vi "Keithley 2002 T-Coup Config.vi"(0 "GPIB address":string="16", 1 "reference (off:0)":u16(ring) items=["off", "set reference value"], 2 "reference value (degs)":dbl format="%^.2e", 3 "T-couple type (J:0)":u16(ring) items=["J thermocouples", "T thermocouples", "K thermocouples", "E thermocouples", "R thermocouples", "S thermocouples", "B thermocouples", "B thermocouples"], 4 "simulated temp. (degs)":dbl=23.0 min=0.0 max=323.0 format="%^.2e", 5 "integration time (0:auto)":u16(ring) items=["automatic", "automatic once", "set to minimum", "set to maximum", "set aperature value", "set NPLC value"], 6 "real coefficient":dbl=0.01 min=-0.09999 max=0.09999 format="%^.2e", 7 "integ. value":dbl=0.01667 format="%^.2e", 8 "real offset":dbl=0.01 min=-0.09999 max=0.09999 format="%^.2e", 9 "resolution (5.5 digits:4)":u16(ring)=4 items=["auto resolution", "auto resolution once", "3.5 digits", "4.5 digits", "5.5 digits", "6.5 digits"], 11 "error in":T1, 12 "digital filter (off:0)":u16(ring) items=["off", "auto filter", "auto filter once", "moving filter", "repeating filter"], 13 "dig. filter count":dbl=10.0 min=1.0 max=100.0 step=1.0 format="%^.2e", 14 "temp (celsius:0)":u16(ring) items=["Celsius", "Fahrenheit", "Kelvin"]) -> (15 "error out":T1)   [LabVIEW 2020]
doc: "This VI is used to configure the settings for the thermo-couple temperature measurements. The instrument can be in any mode when this VI is run. The settings will go into effect and the instrument will go into the Temperature mode."
panel:
  in  "R-junction #":dbl=1.0 min=1.0 max=5.0
  in  "R-junction type":bool=TRUE
  # "simulated\nreal"
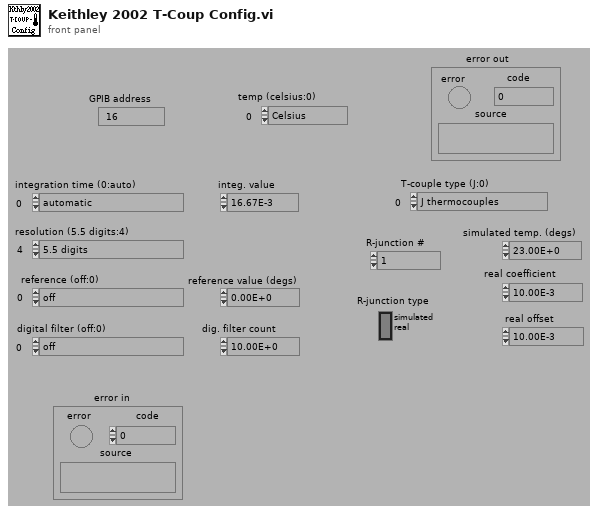
[diagram p1: front panel]
types:
  T1 = cluster{"error":bool, "code":i32, "source":string}
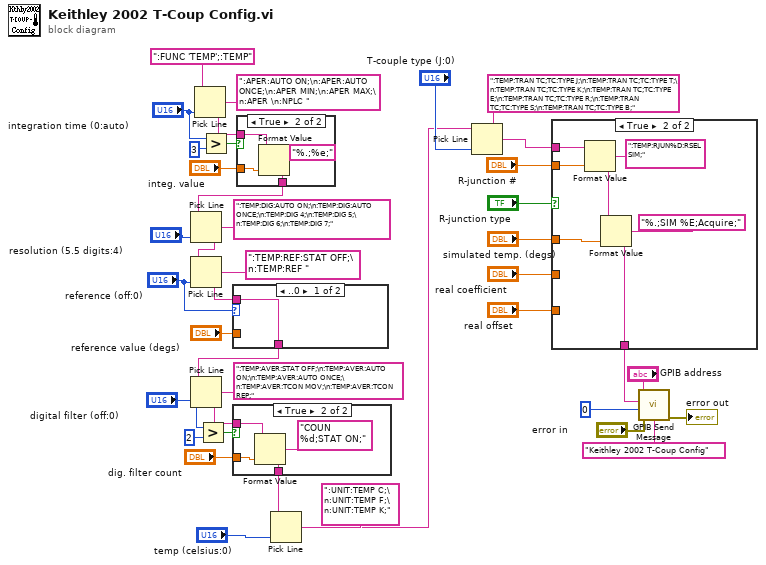
[diagram p0: block diagram]
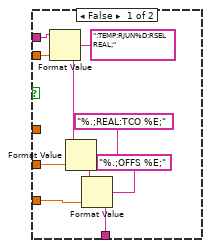
[diagram p2: hidden frame]
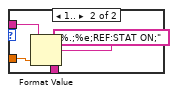
[diagram p4: hidden frame]
diagram:
  n1 = Pick Line(string ("")=":FUNC 'TEMP';:TEMP", multi-line string=":APER:AUTO ON;\n:APER:AUTO ONCE;\n:APER MIN;\n:APER MAX;\n:APER \n:NPLC ", line index="integration time (0:auto)") -> (output string=w34:string)
  n2 = Greater?(x="digital filter (off:0)", y=2) -> (0:w22:bool)
  n3 = Greater?(x="integration time (0:auto)", y=3) -> (0:w35:bool)
  n4 = case shown="True" w35 {
    tunnel: "integ. value" -> [_ w44]
    tunnel: w34 -> [w41 w43]
    tunnel: [w41 w42] -> w14
    frame False {
    }
    frame True {
      n5 = Format Value(string ("")=w43, format string="%.;%e;", value (0)=w44) -> (output string=w42:string)
    }
  }
  n6 = Pick Line(string ("")=w14, multi-line string=":TEMP:DIG:AUTO ON;\n:TEMP:DIG:AUTO ONCE;\n:TEMP:DIG 4;\n:TEMP:DIG 5;\n:TEMP:DIG 6;\n:TEMP:DIG 7;", line index="resolution (5.5 digits:4)") -> (output string=w28:string)
  n7 = Pick Line(string ("")=w28, multi-line string=":TEMP:REF:STAT OFF;\n:TEMP:REF ", line index="reference (off:0)") -> (output string=w31:string)
  n8 = case shown="..0" "reference (off:0)" {
    tunnel: "reference value (degs)" -> [_ w50]
    tunnel: w31 -> [w46 w49]
    tunnel: [w46 w47] -> w15
    frame ..0 {
    }
    frame 1.. {
      n9 = Format Value(string ("")=w49, format string="%.;%e;REF:STAT ON;", value (0)=w50) -> (output string=w47:string)
    }
  }
  n10 = Pick Line(string ("")=w15, multi-line string=":TEMP:AVER:STAT OFF;\n:TEMP:AVER:AUTO ON;\n:TEMP:AVER:AUTO ONCE;\n:TEMP:AVER:TCON MOV;\n:TEMP:AVER:TCON REP;", line index="digital filter (off:0)") -> (output string=w25:string)
  n11 = case shown="True" w22 {
    tunnel: "dig. filter count" -> [_ w55]
    tunnel: w25 -> [w51 w54]
    tunnel: [w51 w53] -> w3
    frame False {
    }
    frame True {
      n12 = Format Value(string ("")=w54, format string="COUN %d;STAT ON;", value (0)=w55) -> (output string=w53:string)
    }
  }
  n13 = Pick Line(string ("")=w3, multi-line string=":UNIT:TEMP C;\n:UNIT:TEMP F;\n:UNIT:TEMP K;", line index="temp (celsius:0)") -> (output string=w1:string)
  n14 = Pick Line(string ("")=w1, multi-line string=":TEMP:TRAN TC;TC:TYPE J;\n:TEMP:TRAN TC;TC:TYPE T;\n:TEMP:TRAN TC;TC:TYPE K;\n:TEMP:TRAN TC;TC:TYPE E;\n:TEMP:TRAN TC;TC:TYPE R;\n:TEMP:TRAN TC;TC:TYPE S;\n:TEMP:TRAN TC;TC:TYPE B;", line index="T-couple type (J:0)") -> (output string=w10:string)
  n15 = case shown="True" "R-junction type" {
    tunnel: w10 -> [w59 w72]
    tunnel: "simulated temp. (degs)" -> [_ w69]
    tunnel: "real coefficient" -> [w63 _]
    tunnel: "real offset" -> [w62 _]
    tunnel: "R-junction #" -> [w60 w71]
    tunnel: [w56 w68] -> w5
    frame False {
      n16 = Format Value(string ("")=w59, format string=":TEMP:RJUN%D:RSEL REAL;", value (0)=w60) -> (output string=w57:string)
      n17 = Format Value(string ("")=w57, format string="%.;REAL:TCO %E;", value (0)=w63) -> (output string=w64:string)
      n18 = Format Value(string ("")=w64, format string="%.;OFFS %E;", value (0)=w62) -> (output string=w56:string)
    }
    frame True {
      n19 = Format Value(string ("")=w72, format string=":TEMP:RJUN%D:RSEL SIM;", value (0)=w71) -> (output string=w70:string)
      n20 = Format Value(string ("")=w70, format string="%.;SIM %E;Acquire;", value (0)=w69) -> (output string=w68:string)
    }
  }
  n21 = call "GPIB Send Message.vi"("address string"="GPIB address", "write buffer"=w5, "source"="Keithley 2002 T-Coup Config", "write mode (set END:0)"=0, "error in"="error in") -> ("error out"=→"error out":T1)  [unwired: 2 in, 2 out]
